vi "Arduino_Connect.vi"(8 "error in (no error)":errorcluster, 9 "SearchCommand":string, 10 "Baud Rate":u16(ring)=57600 items=["57600"=57600, "9600"=9600], 11 "Arduino_Core in":refnum<class "Arduino_Core.lvclass">) -> (0 "error out":errorcluster, 3 "Arduino_Core out":refnum<class "Arduino_Core.lvclass">)   [LabVIEW 2013, in "Arduino_Core.lvclass"]
uses:
  Arduino_Core.lvclass
  Arduino_Core.lvclass/Arduino_Core.ctl
  <vilib>/Instr/_visa.llb/VISA Configure Serial Port (Instr).vi
panel:
  out "Port":string
  out "portVisa":refnum<visa-resource-name>
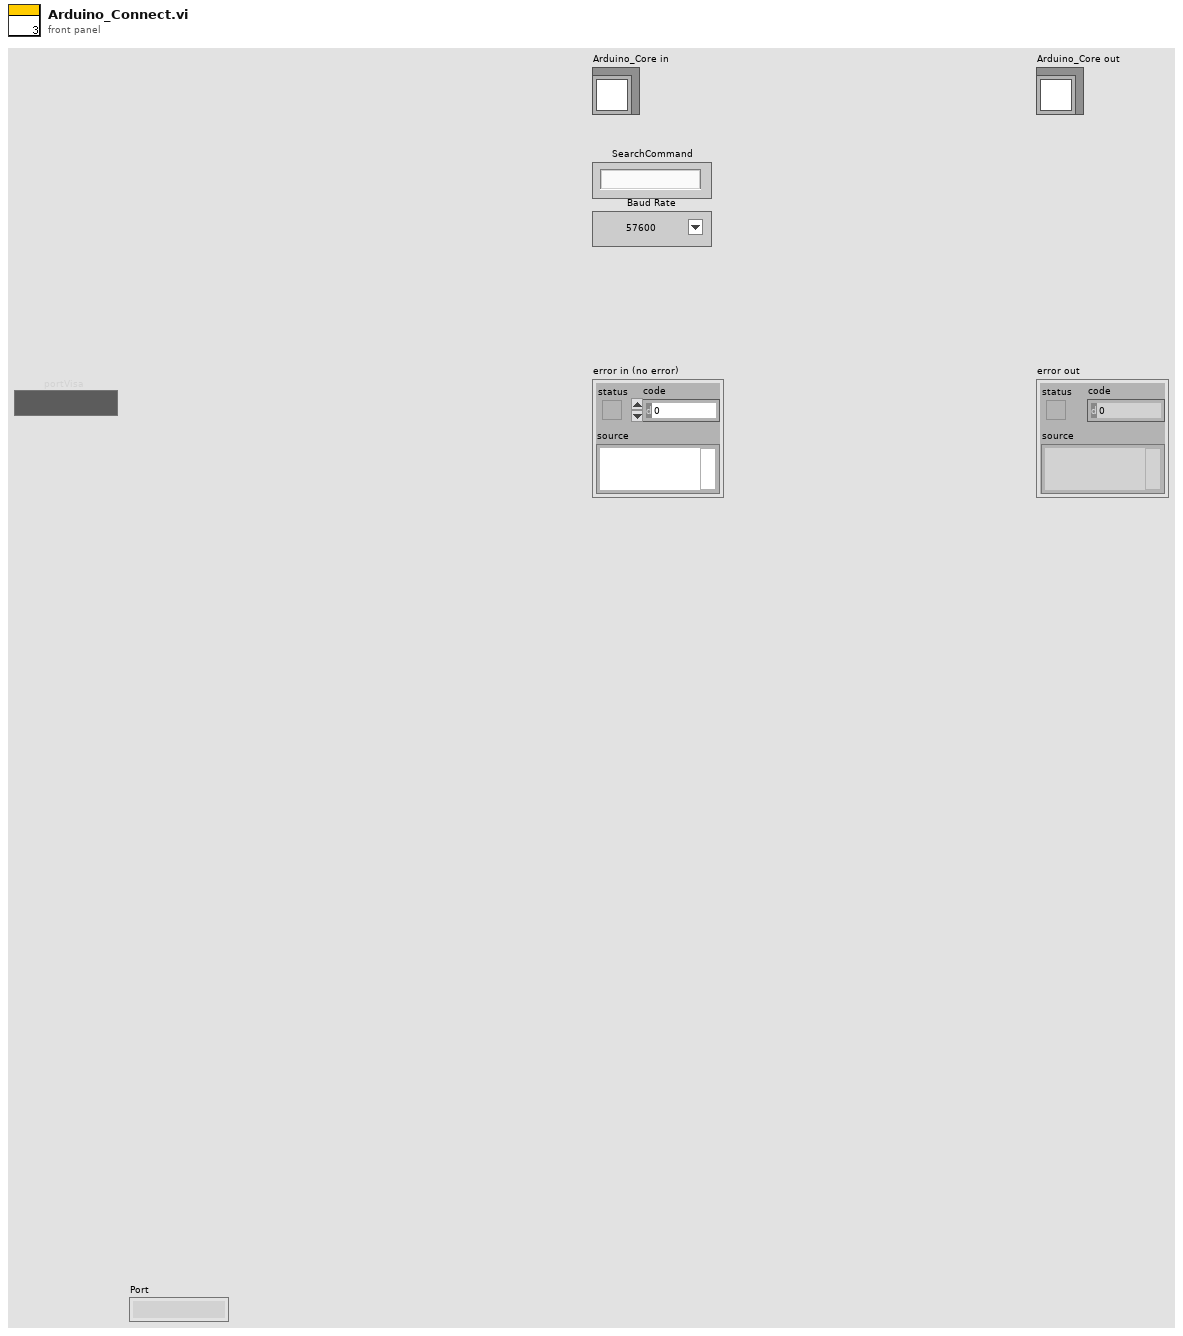
[diagram p1: front panel]
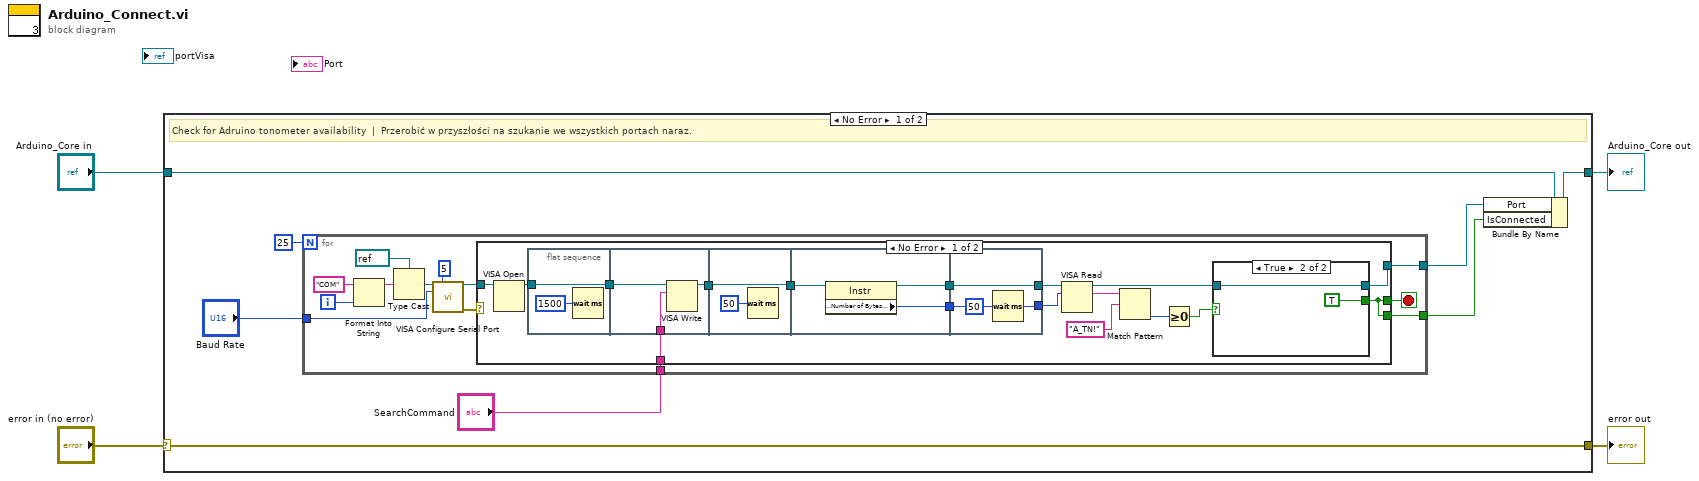
[diagram p0: block diagram]
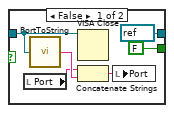
[diagram p2: hidden frame]
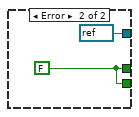
[diagram p3: hidden frame]
diagram:
  n1 = case shown="No Error" "error in (no error)" {
    selector: "error in (no error)" -> [w12 w67]
    tunnel: [w12 w67] -> w3
    tunnel: [w7 w66] -> w1
    tunnel: "Arduino_Core in" -> [w8 w66]
    frame No Error {
      # "Check for Adruino tonometer availability  |  Przerobić w przyszłości na szukanie we wszystkich portach naraz."
      n2 = for {
        N: 25 -> [_]
        tunnel: "Baud Rate" -> [w16]
        tunnel: "SearchCommand" -> [w15]
        tunnel: [w14] -> w6
        tunnel: [w13] -> w5
        i -> [w25]
        stop <- w24 stop-if-true
        n3 = Format Into String(initial string="COM", w25) -> (resulting string=w19:string)  [unwired: 2 in, 1 out]
        n4 = Type Cast(type=refnum<visa-resource-name> refnum ("portVisa"), x=w19) -> (*(type *) &x=w17:refnum<visa-resource-name>)
        n5 = call-poly "VISA Configure Serial Port"("VISA resource name"=w17, "timeout (10sec)"=u32 5, "baud rate (9600)"=w16) -> ("VISA resource name out"=w21:refnum<visa-resource-name>, "error out"=w20:errorcluster)  [unwired: 11 in]
        n6 = case shown="No Error" w20 {
          tunnel: w21 -> [w39 _]
          tunnel: [w26 w64] -> w24
          tunnel: w15 -> [w28 _]
          tunnel: [w27 refnum<visa-resource-name> refnum ("VISA resource name out")] -> w14
          tunnel: [w26 w64] -> w13
          frame No Error {
            n7 = VISA Open(VISA resource name=w39) -> (VISA resource name=w38:refnum<visa-resource-name>)  [unwired: 4 in, 1 out]
            n8 = flat-sequence {
              tunnel: w38 -> [w52]
              tunnel: [w52] -> w37
              tunnel: [w55] -> w40
              tunnel: w37 -> [w54]
              tunnel: w28 -> [w53]
              tunnel: [w57] -> w42
              tunnel: w40 -> [w57]
              tunnel: w42 -> [w60]
              tunnel: [w59] -> w36
              tunnel: [w58] -> w35
              tunnel: w36 -> [w62]
              tunnel: w35 -> [w61]
              tunnel: [w62] -> w34
              tunnel: [w61] -> w33
              frame #0 {
                n9 = Wait (ms)(milliseconds to wait=u32 1500) -> ()  [unwired: 1 out]
              }
              frame #1 {
                n10 = VISA Write(VISA resource name=w54, write buffer=w53) -> (VISA resource name out=w55:refnum<visa-resource-name>)  [unwired: 1 in, 2 out]
              }
              frame #2 {
                n11 = Wait (ms)(milliseconds to wait=u32 50) -> ()  [unwired: 1 out]
              }
              frame #3 {
                n12 = property class="Instr"(reference=w60) -> (reference out=w59:refnum<visa-resource-name>, "Serial Settings:Number of Bytes at Serial Port"=w58:u32)  [unwired: 1 in, 1 out]
              }
              frame #4 {
                n13 = Wait (ms)(milliseconds to wait=u32 50) -> ()  [unwired: 1 out]
              }
            }
            n14 = VISA Read(VISA resource name=w34, byte count=w33) -> (VISA resource name out=w41:refnum<visa-resource-name>, read buffer=w31:string)  [unwired: 1 in, 2 out]
            n15 = Match Pattern(string=w31, regular expression="A_TN!") -> (offset past match=w30:i32)  [unwired: 1 in, 3 out]
            n16 = Greater Or Equal To 0?(x=w30) -> (x >= 0?=w29:bool)
            n17 = case shown="True" w29 {
              tunnel: w41 -> [w47 w49]
              tunnel: [FALSE TRUE] -> w26
              tunnel: [refnum<visa-resource-name> refnum ("VISA resource name out") w49] -> w27
              frame False {
                n18 = local read "Port"() -> (w45:string)
                n19 = call "PortToString.vi"("portVisa"=w47) -> ("Port"=w46:string)
                n20 = VISA Close(VISA resource name=w47) -> ()  [unwired: 1 in, 1 out]
                n21 = Concatenate Strings(w45, w46) -> (w44:string)
                n22 = local write "Port"(w44) -> ()
              }
              frame True {
              }
            }
          }
          frame Error {
            w64 = FALSE
          }
        }
      }
      n23 = Bundle By Name(cluster=w8, "Port"=w6, "IsConnected"=w5) -> (w7:refnum<class "Arduino_Core.lvclass">)
    }
    frame Error {
    }
  }
  "error out" <- w3
  "Arduino_Core out" <- w1
